vi "Tosca-Parse Application Args.vi"(7 "App.Args":string[](array[string])) -> (4 "config":string, 6 "rigname":string, 8 "rignum":i32, 10 "title":string)   [LabVIEW 2020]
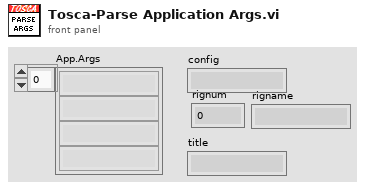
[diagram p1: front panel]
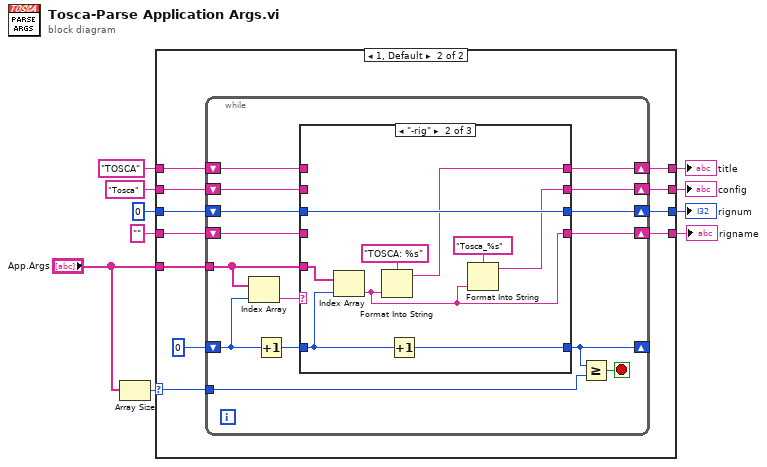
[diagram p0: block diagram]
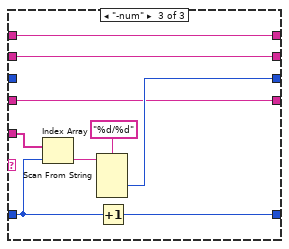
[diagram p4: hidden frame]
diagram:
  n1 = Array Size(array="App.Args") -> (size(s)=w9:i32)
  n2 = case shown="1, Default" w9 {
    selector: w9 -> [_ w23]
    tunnel: "App.Args" -> [_ w24]
    tunnel: "TOSCA" ("title") -> [w14 w22]
    tunnel: "Tosca" ("config") -> [w13 w21]
    tunnel: [w14 w20] -> w5
    tunnel: [w13 w19] -> w4
    tunnel: 0 ("rignum") -> [w12 w18]
    tunnel: [w12 w17] -> w3
    tunnel: [w11 w16] -> w2
    tunnel: "" ("config") -> [w11 w15]
    frame 0 {
    }
    frame 1, Default {
      n3 = while {
        shift-right: [w36] -> _
        shift-left: 0 -> [w39]
        tunnel: w24 -> [w38]
        tunnel: w23 -> [w35]
        shift-right: [w33] -> w20
        shift-left: w22 -> [w32]
        shift-right: [w31] -> w19
        shift-left: w21 -> [w30]
        shift-right: [w29] -> w17
        shift-left: w18 -> [w28]
        shift-right: [w27] -> w16
        shift-left: w15 -> [w26]
        stop <- w34 stop-if-true
        n4 = Index Array(array=w38, index=w39) -> (element=w40:string)
        n5 = Increment(x=w39) -> (x+1=w37:i32)
        n6 = case shown="\"-rig\"" w40 {
          tunnel: w37 -> [w45 w54 w63]
          tunnel: w38 -> [_ w53 w62]
          tunnel: [w45 w52 w61] -> w36
          tunnel: [w44 w48 w58] -> w33
          tunnel: w32 -> [w44 _ w58]
          tunnel: [w43 w47 w57] -> w31
          tunnel: w30 -> [w43 _ w57]
          tunnel: [w42 w49 w56] -> w29
          tunnel: w28 -> [w42 w49 _]
          tunnel: [w41 w46 w55] -> w27
          tunnel: w26 -> [w41 _ w55]
          frame "", Default {
          }
          frame "-rig" {
            n7 = Index Array(array=w53, index=w54) -> (element=w46:string)
            n8 = Format Into String(format string="TOSCA: %s", w46) -> (resulting string=w48:string)  [unwired: 2 in, 1 out]
            n9 = Increment(x=w54) -> (x+1=w52:i32)
            n10 = Format Into String(format string="Tosca_%s", w46) -> (resulting string=w47:string)  [unwired: 2 in, 1 out]
          }
          frame "-num" {
            n11 = Index Array(array=w62, index=w63) -> (element=w60:string)
            n12 = Scan From String(format string="%d/%d", input string=w60) -> (output 1=w56:i32)  [unwired: 5 in, 3 out]
            n13 = Increment(x=w63) -> (x+1=w61:i32)
          }
        }
        n14 = Greater Or Equal?(x=w36, y=w35) -> (x >= y?=w34:bool)
      }
    }
  }
  "title" <- w5
  "config" <- w4
  "rignum" <- w3
  "rigname" <- w2
